vi "Save_Init.vi"(2 "error in":errorcluster, 3 "Init outp register 2 (8-13)":bool[](array[boolean])=[FALSE, FALSE, FALSE, FALSE, FALSE, FALSE], 4 "Init outp register 1 (2-7)":bool[](array[boolean])=[FALSE, FALSE, FALSE, FALSE, FALSE, FALSE], 5 "Filename (.ini)":string="Config_Ver_1\\pulse_sequence.ini") -> (0 "error out":errorcluster)   [LabVIEW 2021]
uses:
  Pulse_Sequence_Global.vi
  <vilib>/Utility/config.llb/Write Key (Boolean).vi
  <vilib>/Utility/config.llb/NI_LVConfig.lvlib
panel:
  # "Remember that config files are .ini, \nconfig file will be save in ...\\Config_Files\\(filename).ini"
  # "One can easily add files into folder placed inside ...\\Config_Files\\ (folder)\nby writing Filename as (folder)\\(filename).ini, but firstly one have to manualy\ncreate that folder"
  # "All used channels should be specified here"
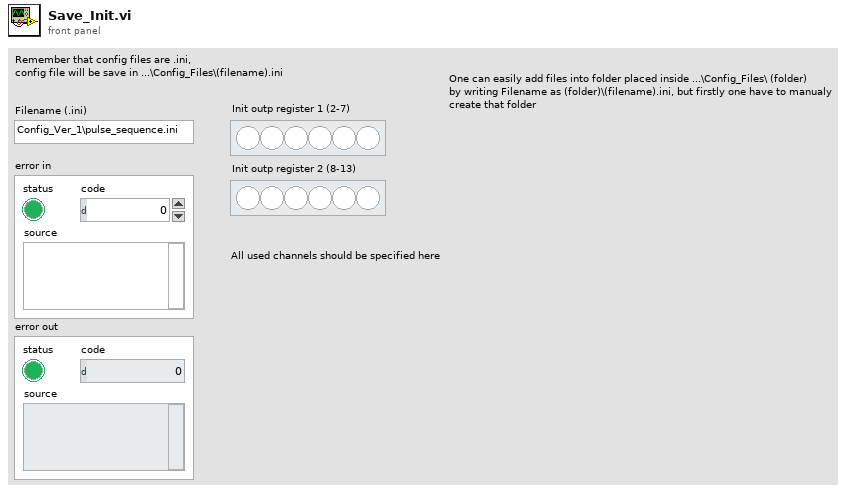
[diagram p1: front panel]
types:
  T1 = typedef "NI_LVConfig.lvlib/Config Data RefNum.ctl" = refnum<k1>
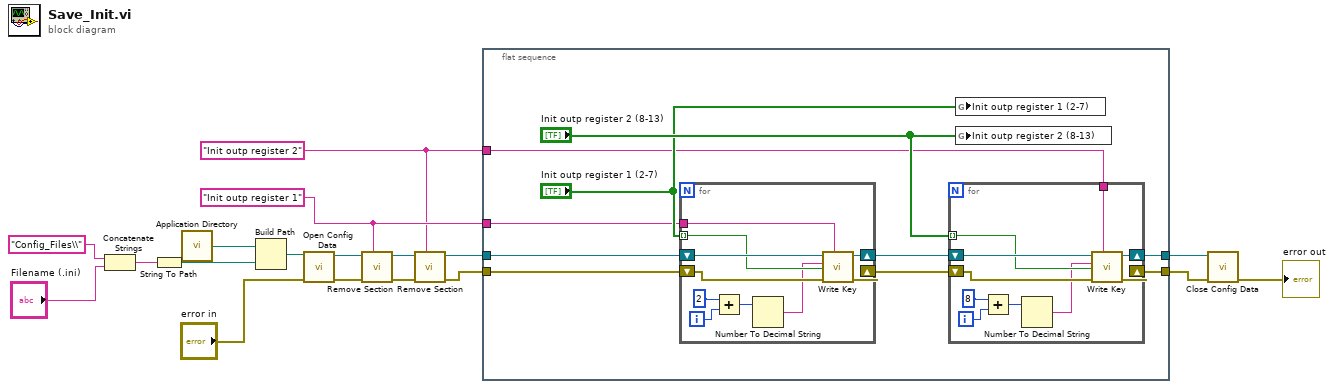
[diagram p0: block diagram]
diagram:
  w2 = "Init outp register 1" ("section")
  w1 = "Init outp register 2" ("section")
  n1 = Concatenate Strings("Config_Files\\" ("string"), "Filename (.ini)") -> (w12:string)
  n2 = String To Path(string=w12) -> (path=w15:path)
  n3 = call <vilib>:"Application Directory.vi"() -> ("Application Directory"=w18:path)
  n4 = Build Path(base path=w18, name or relative path=w15) -> (appended path=w17:path)
  n5 = call <vilib>:"Open Config Data.vi"("error in (no error)"="error in", "configuration file path"=w17) -> ("error out"=w8:errorcluster, "refnum"=w7:T1)  [unwired: 7 in, 1 out]
  n6 = call <vilib>:"Remove Section.vi"("section"=w2, "error in (no error)"=w8, "refnum"=w7) -> ("error out"=w6:errorcluster, "refnum out"=w3:T1)  [unwired: 6 in, 1 out]
  n7 = call <vilib>:"Remove Section.vi"("section"=w1, "error in (no error)"=w6, "refnum"=w3) -> ("error out"=w5:errorcluster, "refnum out"=w4:T1)  [unwired: 6 in, 1 out]
  n8 = flat-sequence {
    tunnel: w5 -> [w28]
    tunnel: w4 -> [w27]
    tunnel: [w24] -> w11
    tunnel: [w23] -> w10
    tunnel: w1 -> [w20]
    tunnel: w2 -> [w19]
    frame #0 {
      n9 = for {
        tunnel: "Init outp register 1 (2-7)" -> [w42] mode=indexing
        shift-right: [w47] -> w26
        shift-left: w28 -> [w45]
        shift-right: [w46] -> w25
        shift-left: w27 -> [w48]
        tunnel: w19 -> [w39]
        i -> [w44]
        n10 = Add(x=2, y=w44) -> (x+y=w41:i32)
        n11 = Number To Decimal String(number=w41) -> (decimal integer string=w40:string)  [unwired: 1 in]
        n12 = call-poly <vilib>:"Write Key.vi"("section"=w39, "error in (no error)"=w45, "value"=w42, "key"=w40, "refnum"=w48) -> ("error out"=w47:errorcluster, "refnum out"=w46:T1)  [unwired: 4 in, 1 out]
      }
      n13 = for {
        tunnel: "Init outp register 2 (8-13)" -> [w32] mode=indexing
        shift-right: [w37] -> w24
        shift-left: w26 -> [w35]
        shift-right: [w36] -> w23
        shift-left: w25 -> [w38]
        tunnel: w20 -> [w29]
        i -> [w34]
        n14 = Add(x=8, y=w34) -> (x+y=w31:i32)
        n15 = Number To Decimal String(number=w31) -> (decimal integer string=w30:string)  [unwired: 1 in]
        n16 = call-poly <vilib>:"Write Key.vi"("section"=w29, "error in (no error)"=w35, "value"=w32, "key"=w30, "refnum"=w38) -> ("error out"=w37:errorcluster, "refnum out"=w36:T1)  [unwired: 4 in, 1 out]
      }
      n17 = global write "Pulse_Sequence_Global.vi" "Init outp register 1 (2-7)"("Init outp register 1 (2-7)") -> ()
      n18 = global write "Pulse_Sequence_Global.vi" "Init outp register 2 (8-13)"("Init outp register 2 (8-13)") -> ()
    }
  }
  n19 = call <vilib>:"Close Config Data.vi"("error in (no error)"=w11, "refnum"=w10) -> ("error out"=→"error out":errorcluster)  [unwired: 8 in, 1 out]
